vi "Autonomous Independent.vi"   [LabVIEW 2014]
doc: "This VI is called when autonomous begins, and will automatically be terminated when autonomous ends. You can carry out timed or sensor driven robot movement independently without needing to return to the caller."
uses:
  <vilib>/Rock Robotics/Network Tables/SD Write Numeric Array.vi
  <vilib>/Rock Robotics/WPI/RobotDrive/WPI_RobotDriveMecanumDrive_Cartesian.vi
panel:
  # "Be sure to right-click and choose Data Operations>>Make Current Value default if you want to save the array values with the VI"
types:
  T1 = typedef "WPI_RobotDriveDevRef.ctl" = cluster{"DevStatus":errorcluster, "Motors[]":T2[], "Square Inputs":bool, "Max Output":dbl}
  T2 = typedef "WPI_MotorControlDeviceRef.ctl" = cluster{"DeviceStatus":errorcluster, "Type":T3, "PWM":cluster{"Controller":T4, "PWM Channel":T5, "DeadBand":T6}, "CAN":cluster{"Device Number":u8, "Control Mode":T7, "Semaphore":T8, "Max Vout":dbl, "TalonSRX Control Mode":T9}, "Invert":bool, "TransformRef":T10, "InvTransformRef":T10}
  T3 = typedef "WPI_MotorControlType.ctl" = enum16{"PWM", "CAN", "CANTalonSRX"}
  T4 = typedef "FPGA_TypedefDigitalModule.ctl" = enum16{"Controller 1"}
  T5 = typedef "FPGA_DIOPWMChannel.ctl" = enum8{"PWM 0", "PWM 1", "PWM 2", "PWM 3", "PWM 4", "PWM 5", "PWM 6", "PWM 7", "PWM 8", "PWM 9", "PWM MXP 0", "PWM MXP 1", "PWM MXP 2", "PWM MXP 3", "PWM MXP 4", "PWM MXP 5", "PWM MXP 6", "PWM MXP 7", "PWM MXP 8", "PWM MXP 9", "Invalid"}
  T6 = typedef "WPI_PWMDeadband.ctl" = cluster{"Name":string, "maxPositivePwm":i32, "minPositivePwm":i32, "centerPwm":i32, "maxNegativePwm":i32, "minNegativePwm":i32, "angularRange":u16}
  T7 = typedef "WPI_CANJaguar_ControlMode.ctl" = enum8{"Percent VBus", "Current", "Speed", "Position", "Voltage"}
  T8 = typedef "Semaphore RefNum" = refnum<k1>
  T9 = typedef "WPI_CANTalonSRX_APIControlMode.ctl" = enum8{"Percent VBus", "Speed", "Position", "Slave", "Unchanged / Invalid"}
  T10 = typedef "WPI_PWMTransform_ConPane.ctl" = refnum<vi>
  T11 = typedef "WPI_JoystickDevRef.ctl" = cluster{"Device":T12}
  T12 = typedef "WPI_JoystickDeviceEnum.ctl" = enum16{"USB 0", "USB 1", "USB 2", "USB 3", "USB 4", "USB 5"}
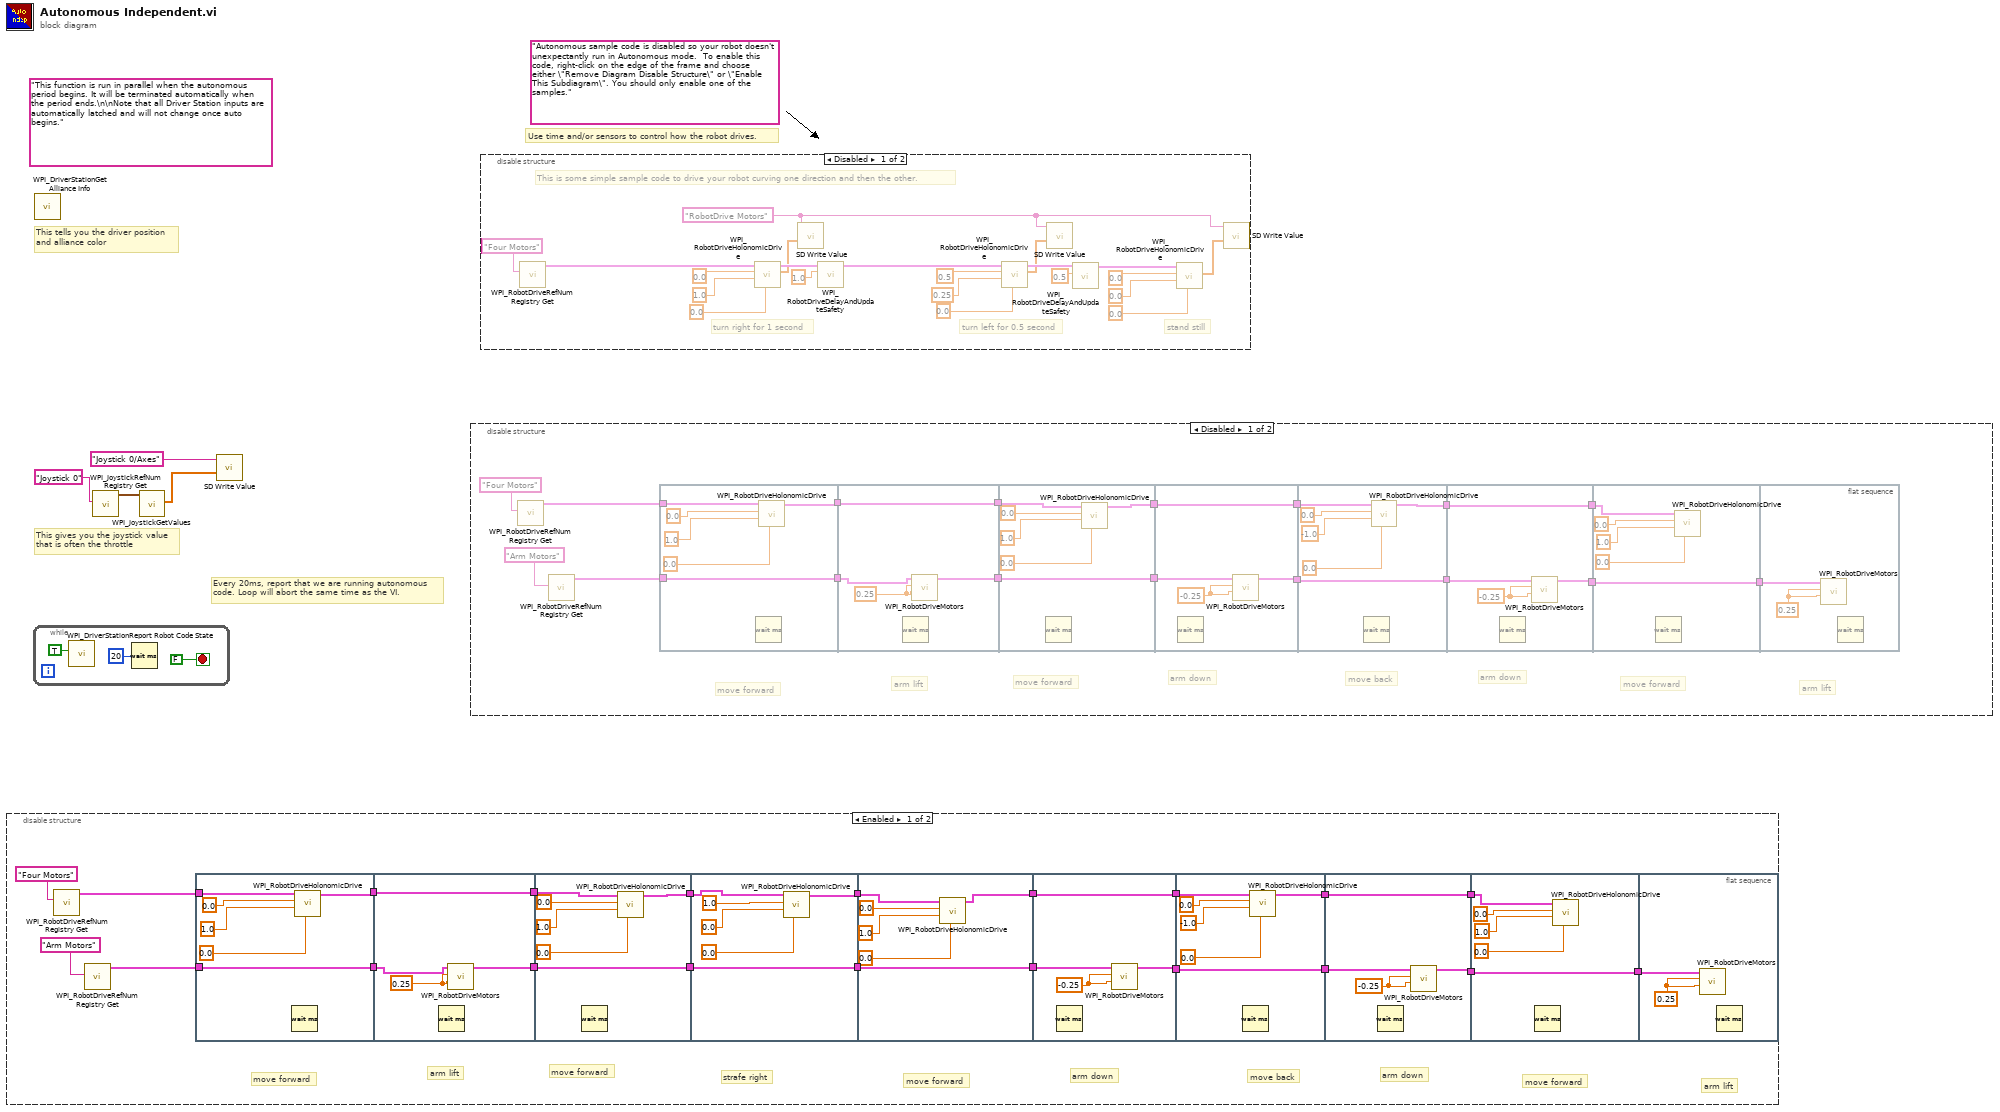
[diagram p0: block diagram]
diagram:
  (unwired) "Autonomous sample code is disabled so your robot doesn't unexpectantly run in Autonomous mode.  To enable this code, right-click on the edge of the frame and choose either \"Remove Diagram Disable Structure\" or \"Enable This Subdiagram\". You should only enable one of the samples."
  (unwired) "This function is run in parallel when the autonomous period begins. It will be terminated automatically when the period ends.\n\nNote that all Driver Station inputs are automatically latched and will not change once auto begins."
  # "Every 20ms, report that we are running autonomous\ncode. Loop will abort the same time as the VI."
  # "This gives you the joystick value\nthat is often the throttle"
  # "Use time and/or sensors to control how the robot drives."
  # "This tells you the driver position\nand alliance color"
  n1 = disable-structure shown="Enabled" {
    frame Enabled {
      # "move forward"
      # "strafe right"
      # "arm lift"
      # "move forward"
      # "arm down"
      # "move back"
      # "arm down"
      # "move forward"
      # "arm lift"
      # "move forward"
      n2 = call <vilib>:"WPI_RobotDriveRefNum Registry Get.vi"("refnum name"="Four Motors") -> ("RobotDriveDevRef"=w13:T1)  [unwired: 1 in, 9 out]
      n3 = call <vilib>:"WPI_RobotDriveRefNum Registry Get.vi"("refnum name"="Arm Motors") -> ("RobotDriveDevRef"=w11:T1)  [unwired: 9 in, 1 out]
      n4 = flat-sequence {
        tunnel: w13 -> [w29]
        tunnel: [w30] -> w25
        tunnel: w11 -> [w31]
        tunnel: [w31] -> w24
        tunnel: [w35] -> w23
        tunnel: w25 -> [w35]
        tunnel: w24 -> [w34]
        tunnel: [w33] -> w22
        tunnel: w23 -> [w41]
        tunnel: [w40] -> w10
        tunnel: [w39] -> w9
        tunnel: w22 -> [w39]
        tunnel: w10 -> [w43]
        tunnel: [w42] -> w8
        tunnel: w9 -> [w47]
        tunnel: [w47] -> w6
        tunnel: w8 -> [w49]
        tunnel: [w48] -> w7
        tunnel: w6 -> [w53]
        tunnel: [w53] -> w5
        tunnel: [w57] -> w21
        tunnel: w7 -> [w57]
        tunnel: [w56] -> w20
        tunnel: w5 -> [w55]
        tunnel: w21 -> [w62]
        tunnel: [w61] -> w19
        tunnel: w20 -> [w60]
        tunnel: [w60] -> w18
        tunnel: [w67] -> w17
        tunnel: w19 -> [w67]
        tunnel: [w66] -> w16
        tunnel: w18 -> [w65]
        tunnel: w17 -> [w72]
        tunnel: [w71] -> w15
        tunnel: w16 -> [w71]
        tunnel: w15 -> [w74]
        frame #0 {
          n5 = Wait (ms)() -> ()  [unwired: 1 in, 1 out]
          n6 = call-poly <vilib>:"WPI_RobotDriveHolonomicDrive.vi"("Rotation"=0.0, "Y"=1.0 ("X axis value"), "X"=0.0 ("X axis value"), "RobotDriveDevRef"=w29) -> ("RobotDriveDevRef"=w30:T1)  [unwired: 5 in, 2 out]
        }
        frame #1 {
          w32 = 0.25
          n7 = Wait (ms)() -> ()  [unwired: 1 in, 1 out]
          n8 = call <vilib>:"WPI_RobotDriveMotors.vi"("RightSpeed"=w32, "LeftSpeed"=w32, "RobotDriveDevRef"=w34) -> ("RobotDriveDevRef"=w33:T1)  [unwired: 6 in, 2 out]
        }
        frame #2 {
          n9 = Wait (ms)() -> ()  [unwired: 1 in, 1 out]
          n10 = call-poly <vilib>:"WPI_RobotDriveHolonomicDrive.vi"("Rotation"=0.0, "Y"=1.0 ("X axis value"), "X"=0.0 ("X axis value"), "RobotDriveDevRef"=w41) -> ("RobotDriveDevRef"=w40:T1)  [unwired: 5 in, 2 out]
        }
        frame #3 {
          n11 = call-poly <vilib>:"WPI_RobotDriveHolonomicDrive.vi"("Rotation"=0.0, "Y"=0.0 ("X axis value"), "X"=1.0 ("X axis value"), "RobotDriveDevRef"=w43) -> ("RobotDriveDevRef"=w42:T1)  [unwired: 5 in, 2 out]
        }
        frame #4 {
          n12 = call-poly <vilib>:"WPI_RobotDriveHolonomicDrive.vi"("Rotation"=0.0, "Y"=1.0 ("X axis value"), "X"=0.0 ("X axis value"), "RobotDriveDevRef"=w49) -> ("RobotDriveDevRef"=w48:T1)  [unwired: 5 in, 2 out]
        }
        frame #5 {
          w54 = -0.25
          n13 = Wait (ms)() -> ()  [unwired: 1 in, 1 out]
          n14 = call <vilib>:"WPI_RobotDriveMotors.vi"("RightSpeed"=w54, "LeftSpeed"=w54, "RobotDriveDevRef"=w55) -> ("RobotDriveDevRef"=w56:T1)  [unwired: 6 in, 2 out]
        }
        frame #6 {
          n15 = Wait (ms)() -> ()  [unwired: 1 in, 1 out]
          n16 = call-poly <vilib>:"WPI_RobotDriveHolonomicDrive.vi"("Rotation"=0.0, "Y"=-1.0 ("X axis value"), "X"=0.0 ("X axis value"), "RobotDriveDevRef"=w62) -> ("RobotDriveDevRef"=w61:T1)  [unwired: 5 in, 2 out]
        }
        frame #7 {
          w64 = -0.25
          n17 = Wait (ms)() -> ()  [unwired: 1 in, 1 out]
          n18 = call <vilib>:"WPI_RobotDriveMotors.vi"("RightSpeed"=w64, "LeftSpeed"=w64, "RobotDriveDevRef"=w65) -> ("RobotDriveDevRef"=w66:T1)  [unwired: 6 in, 2 out]
        }
        frame #8 {
          n19 = Wait (ms)() -> ()  [unwired: 1 in, 1 out]
          n20 = call-poly <vilib>:"WPI_RobotDriveHolonomicDrive.vi"("Rotation"=0.0, "Y"=1.0 ("X axis value"), "X"=0.0 ("X axis value"), "RobotDriveDevRef"=w72) -> ()  [unwired: 5 in, 3 out]
        }
        frame #9 {
          w73 = 0.25
          n21 = call <vilib>:"WPI_RobotDriveMotors.vi"("RightSpeed"=w73, "LeftSpeed"=w73, "RobotDriveDevRef"=w74) -> ()  [unwired: 6 in, 3 out]
          n22 = Wait (ms)() -> ()  [unwired: 1 in, 1 out]
        }
      }
    }
    frame Disabled {
    }
  }
  n23 = while {
    stop <- FALSE stop-if-true
    n24 = call <vilib>:"WPI_DriverStationReport Robot Code State.vi"("Autonomous"=TRUE) -> ()  [unwired: 10 in, 1 out]
    n25 = Wait (ms)(milliseconds to wait=u32 20) -> ()  [unwired: 1 out]
  }
  n26 = call <vilib>:"WPI_DriverStationGet Alliance Info.vi"() -> ()  [unwired: 12 out]
  n27 = call <vilib>:"WPI_JoystickRefNum Registry Get.vi"("refnum name"="Joystick 0") -> ("JoystickDevRef"=w3:T11)  [unwired: 1 in, 9 out]
  n28 = call <vilib>:"WPI_JoystickGetValues.vi"("JoystickDevRef"=w3) -> ("Axes"=w1:dbl[])  [unwired: 6 in, 4 out]
  n29 = call-poly <vilib>:"SD Write Value.vi"("Numeric Array"=w1, "Name"="Joystick 0/Axes") -> ()  [unwired: 8 in, 2 out]
  n30 = disable-structure shown="Disabled" {
    frame Disabled {
      # "arm lift"
      # "move forward"
      # "arm down"
      # "move back"
      # "arm down"
      # "move forward"
      # "arm lift"
      # "move forward"
      n31 = call <vilib>:"WPI_RobotDriveRefNum Registry Get.vi"("refnum name"="Four Motors") -> ("RobotDriveDevRef"=w80:T1)  [unwired: 1 in, 9 out]
      n32 = call <vilib>:"WPI_RobotDriveRefNum Registry Get.vi"("refnum name"="Arm Motors") -> ("RobotDriveDevRef"=w78:T1)  [unwired: 9 in, 1 out]
      n33 = flat-sequence {
        tunnel: w80 -> [w98]
        tunnel: [w99] -> w94
        tunnel: w78 -> [w100]
        tunnel: [w100] -> w93
        tunnel: [w104] -> w92
        tunnel: w94 -> [w104]
        tunnel: w93 -> [w103]
        tunnel: [w102] -> w91
        tunnel: w92 -> [w110]
        tunnel: [w109] -> w90
        tunnel: [w108] -> w89
        tunnel: w91 -> [w108]
        tunnel: [w114] -> w88
        tunnel: w90 -> [w114]
        tunnel: [w113] -> w87
        tunnel: w89 -> [w112]
        tunnel: w88 -> [w119]
        tunnel: [w118] -> w86
        tunnel: w87 -> [w117]
        tunnel: [w117] -> w85
        tunnel: [w124] -> w84
        tunnel: w86 -> [w124]
        tunnel: [w123] -> w83
        tunnel: w85 -> [w122]
        tunnel: w84 -> [w129]
        tunnel: [w128] -> w82
        tunnel: w83 -> [w128]
        tunnel: w82 -> [w131]
        frame #0 {
          n34 = Wait (ms)() -> ()  [unwired: 1 in, 1 out]
          n35 = call-poly <vilib>:"WPI_RobotDriveHolonomicDrive.vi"("Rotation"=0.0, "Y"=1.0 ("X axis value"), "X"=0.0 ("X axis value"), "RobotDriveDevRef"=w98) -> ("RobotDriveDevRef"=w99:T1)  [unwired: 5 in, 2 out]
        }
        frame #1 {
          w101 = 0.25
          n36 = Wait (ms)() -> ()  [unwired: 1 in, 1 out]
          n37 = call <vilib>:"WPI_RobotDriveMotors.vi"("RightSpeed"=w101, "LeftSpeed"=w101, "RobotDriveDevRef"=w103) -> ("RobotDriveDevRef"=w102:T1)  [unwired: 6 in, 2 out]
        }
        frame #2 {
          n38 = Wait (ms)() -> ()  [unwired: 1 in, 1 out]
          n39 = call-poly <vilib>:"WPI_RobotDriveHolonomicDrive.vi"("Rotation"=0.0, "Y"=1.0 ("X axis value"), "X"=0.0 ("X axis value"), "RobotDriveDevRef"=w110) -> ("RobotDriveDevRef"=w109:T1)  [unwired: 5 in, 2 out]
        }
        frame #3 {
          w111 = -0.25
          n40 = Wait (ms)() -> ()  [unwired: 1 in, 1 out]
          n41 = call <vilib>:"WPI_RobotDriveMotors.vi"("RightSpeed"=w111, "LeftSpeed"=w111, "RobotDriveDevRef"=w112) -> ("RobotDriveDevRef"=w113:T1)  [unwired: 6 in, 2 out]
        }
        frame #4 {
          n42 = Wait (ms)() -> ()  [unwired: 1 in, 1 out]
          n43 = call-poly <vilib>:"WPI_RobotDriveHolonomicDrive.vi"("Rotation"=0.0, "Y"=-1.0 ("X axis value"), "X"=0.0 ("X axis value"), "RobotDriveDevRef"=w119) -> ("RobotDriveDevRef"=w118:T1)  [unwired: 5 in, 2 out]
        }
        frame #5 {
          w121 = -0.25
          n44 = Wait (ms)() -> ()  [unwired: 1 in, 1 out]
          n45 = call <vilib>:"WPI_RobotDriveMotors.vi"("RightSpeed"=w121, "LeftSpeed"=w121, "RobotDriveDevRef"=w122) -> ("RobotDriveDevRef"=w123:T1)  [unwired: 6 in, 2 out]
        }
        frame #6 {
          n46 = Wait (ms)() -> ()  [unwired: 1 in, 1 out]
          n47 = call-poly <vilib>:"WPI_RobotDriveHolonomicDrive.vi"("Rotation"=0.0, "Y"=1.0 ("X axis value"), "X"=0.0 ("X axis value"), "RobotDriveDevRef"=w129) -> ()  [unwired: 5 in, 3 out]
        }
        frame #7 {
          w130 = 0.25
          n48 = call <vilib>:"WPI_RobotDriveMotors.vi"("RightSpeed"=w130, "LeftSpeed"=w130, "RobotDriveDevRef"=w131) -> ()  [unwired: 6 in, 3 out]
          n49 = Wait (ms)() -> ()  [unwired: 1 in, 1 out]
        }
      }
    }
    frame Disabled {
    }
  }
  n50 = disable-structure shown="Disabled" {
    frame Disabled {
      w139 = "RobotDrive Motors" ("Name")
      # "This is some simple sample code to drive your robot curving one direction and then the other."
      # "stand still"
      # "turn left for 0.5 second"
      # "turn right for 1 second"
      n51 = call <vilib>:"WPI_RobotDriveRefNum Registry Get.vi"("refnum name"="Four Motors") -> ("RobotDriveDevRef"=w132:T1)  [unwired: 1 in, 9 out]
      n52 = call-poly <vilib>:"WPI_RobotDriveHolonomicDrive.vi"("Rotation"=0.0, "Y"=1.0 ("X axis value"), "X"=0.0 ("X axis value"), "RobotDriveDevRef"=w132) -> ("Motor Values"=w135:dbl[], "RobotDriveDevRef"=w146:T1)  [unwired: 5 in, 1 out]
      n53 = call-poly <vilib>:"SD Write Value.vi"("Numeric Array"=w135, "Name"=w139) -> ()  [unwired: 8 in, 2 out]
      n54 = call <vilib>:"WPI_RobotDriveDelayAndUpdateSafety.vi"("Delay (s)"=1.0, "RobotDriveDevRef"=w146) -> ("RobotDriveDevRef 2"=w145:T1)  [unwired: 8 in, 1 out]
      n55 = call-poly <vilib>:"WPI_RobotDriveHolonomicDrive.vi"("Rotation"=0.0, "Y"=0.25 ("X axis value"), "X"=0.5 ("X axis value"), "RobotDriveDevRef"=w145) -> ("Motor Values"=w134:dbl[], "RobotDriveDevRef"=w144:T1)  [unwired: 5 in, 1 out]
      n56 = call-poly <vilib>:"SD Write Value.vi"("Numeric Array"=w134, "Name"=w139) -> ()  [unwired: 8 in, 2 out]
      n57 = call <vilib>:"WPI_RobotDriveDelayAndUpdateSafety.vi"("Delay (s)"=0.5, "RobotDriveDevRef"=w144) -> ("RobotDriveDevRef 2"=w143:T1)  [unwired: 8 in, 1 out]
      n58 = call-poly <vilib>:"WPI_RobotDriveHolonomicDrive.vi"("Rotation"=0.0 ("X axis value"), "Y"=0.0 ("X axis value"), "X"=0.0 ("X axis value"), "RobotDriveDevRef"=w143) -> ("Motor Values"=w133:dbl[])  [unwired: 5 in, 2 out]
      n59 = call-poly <vilib>:"SD Write Value.vi"("Numeric Array"=w133, "Name"=w139) -> ()  [unwired: 8 in, 2 out]
    }
    frame Disabled {
    }
  }
